vi "sent_to_dds.vi"(8 "inversion selector":T1(ring), 9 "address bits in":u8, 10 "DDS1 input":u8, 11 "DDS0 input":u8) -> ()   [LabVIEW 2010]
uses:
  <vilib>/eio/EIONode/EIONode.xnode
  <vilib>/rvi/eio/nirviEIOImplementation/nirviEIOImplementation.xnode
  <vilib>/rvi/eio/common/nirviEmuClasses.ctl
  <vilib>/rvi/eio/common/nirviEmuTemplateMethod_noerrors.vi
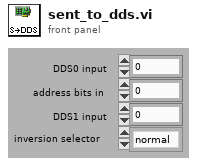
[diagram p1: front panel]
types:
  T1 = enum16{"normal", "x inversed", "y inversed", "x & y inversed"}
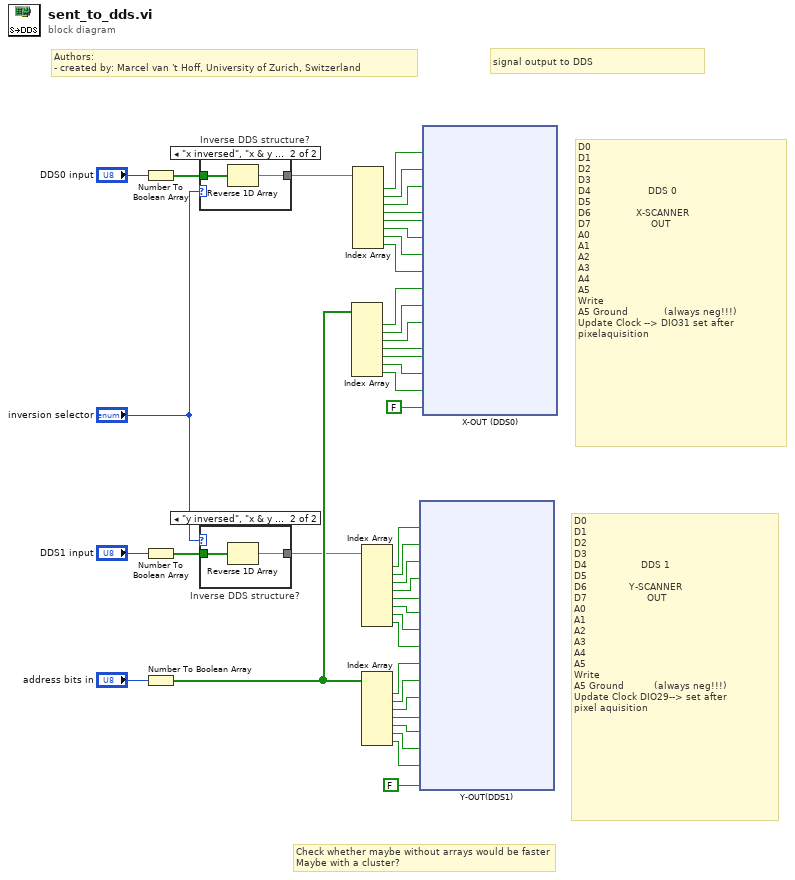
[diagram p0: block diagram]
diagram:
  # "Check whether maybe without arrays would be faster\nMaybe with a cluster?"
  # "D0                                     \nD1\nD2\nD3                        \nD4                  DDS 1\nD5\nD6              Y-SCANNER\nD7                    OUT\nA0\nA1\nA2\nA3\nA4\nA5\nWrite  \nA5 Ground          (always neg!!!)\nUpdate Clock DIO29--> set after \npixel aquisition"
  # "D0                                      \nD1\nD2\nD3                        \nD4                   DDS 0\nD5                  \nD6               X-SCANNER\nD7                    OUT\nA0\nA1\nA2\nA3\nA4\nA5\nWrite\nA5 Ground            (always neg!!!) \nUpdate Clock --> DIO31 set after \npixelaquisition"
  # "Authors: \n- created by: Marcel van 't Hoff, University of Zurich, Switzerland"
  # "signal output to DDS"
  n1 = Number To Boolean Array(number="DDS0 input") -> (Boolean array=w2:bool[])
  n2 = Number To Boolean Array(number="DDS1 input") -> (Boolean array=w5:bool[])
  n3 = Number To Boolean Array(number="address bits in") -> (Boolean array=w16:bool[])
  n4 = case "Inverse DDS structure?" shown="\"x inversed\", \"x & y inversed\"" "inversion selector" {
    tunnel: [w42 w43] -> w1
    tunnel: w2 -> [w42 w44]
    frame Default {
    }
    frame "x inversed", "x & y inversed" {
      n5 = Reverse 1D Array(array=w44) -> (reversed array=w43:bool[])
    }
  }
  n6 = case "Inverse DDS structure?" shown="\"y inversed\", \"x & y inversed\"" "inversion selector" {
    tunnel: [w45 w46] -> w4
    tunnel: w5 -> [w45 w47]
    frame Default {
    }
    frame "y inversed", "x & y inversed" {
      n7 = Reverse 1D Array(array=w47) -> (reversed array=w46:bool[])
    }
  }
  n8 = Index Array(array=w16) -> (element #1=w39:bool, element #2=w38:bool, element #3=w37:bool, element #4=w36:bool, element #5=w35:bool, element #6=w34:bool, element #7=w33:bool)  [unwired: 7 in]
  n9 = Index Array(array=w1) -> (element #1=w32:bool, element #2=w31:bool, element #3=w30:bool, element #4=w29:bool, element #5=w28:bool, element #6=w27:bool, element #7=w26:bool, element #8=w25:bool)  [unwired: 8 in]
  n10 = Index Array(array=w4) -> (element #1=w24:bool, element #2=w23:bool, element #3=w22:bool, element #4=w21:bool, element #5=w20:bool, element #6=w19:bool, element #7=w18:bool, element #8=w17:bool)  [unwired: 8 in]
  n11 = Index Array(array=w16) -> (element #1=w15:bool, element #2=w14:bool, element #3=w13:bool, element #4=w12:bool, element #5=w11:bool, element #6=w10:bool, element #7=w9:bool)  [unwired: 7 in]
  n12 = xnode "Y-OUT(DDS1)"("Connector3/DIO0"=w24, "Connector3/DIO1"=w23, "Connector3/DIO2"=w22, "Connector3/DIO3"=w21, "Connector3/DIO4"=w20, "Connector3/DIO5"=w19, "Connector3/DIO6"=w18, "Connector3/DIO7"=w17, "Connector3/DIO16"=w15, "Connector3/DIO17"=w14, "Connector3/DIO18"=w13, "Connector3/DIO19"=w12, "Connector3/DIO20"=w11, "Connector3/DIO37"=w10, "Connector3/DIO26"=w9, "Connector3/DIO36"=FALSE) -> ()  [unwired: 16 in, 16 out]
  n13 = xnode "X-OUT (DDS0)"("Connector3/DIO15"=w32, "Connector3/DIO14"=w31, "Connector3/DIO13"=w30, "Connector3/DIO12"=w29, "Connector3/DIO11"=w28, "Connector3/DIO10"=w27, "Connector3/DIO9"=w26, "Connector3/DIO8"=w25, "Connector3/DIO21"=w39, "Connector3/DIO22"=w38, "Connector3/DIO23"=w37, "Connector3/DIO24"=w36, "Connector3/DIO25"=w35, "Connector3/DIO35"=w34, "Connector3/DIO27"=w33, "Connector3/DIO34"=FALSE) -> ()  [unwired: 16 in, 16 out]
